vi "Storage Factory.vi"(10 "Format":T1, 11 "Config Path":path) -> (2 "Storage":refnum<class "Config Storage.lvclass">)   [LabVIEW 2020, in "VolatusConfig.lvlib"]
uses:
  VolatusConfig.lvlib
  Config Format.ctl
  lv-cdm/CDM-Config/Config Storage/Config Storage.lvclass
  lv-cdm/CDM-Config/Config-JSON/Config-JSON.lvclass
  C:/dev/lv20CE/relink/lv-cdm/CDM-Config/Config Storage/Config Storage.lvclass
  lv-cdm/CDM-Config/Config-INI/Config-INI.lvclass
  lv-cdm/CDM-Config/Config-Sqlite/Config-Sqlite.lvclass
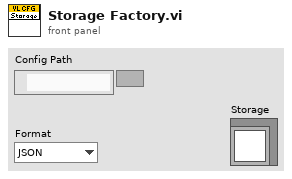
[diagram p1: front panel]
types:
  T1 = typedef "VolatusConfig.lvlib/Config Format.ctl" = enum16{"JSON", "INI", "SQLite"}
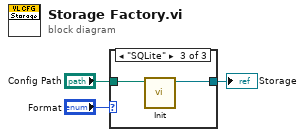
[diagram p0: block diagram]
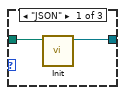
[diagram p2: hidden frame]
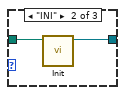
[diagram p3: hidden frame]
diagram:
  n1 = case shown="\"SQLite\"" "Format" {
    tunnel: "Config Path" -> [w5 w7 w9]
    tunnel: [w4 w6 w8] -> w1
    frame "JSON" {
      n2 = call "Init.vi"("Path"=w5) -> ("Config-JSON out"=w4:refnum<class "Config-JSON.lvclass">)  [unwired: 9 in, 1 out]
    }
    frame "INI" {
      n3 = call "Init.vi"("INI Path"=w7) -> ("Config-INI out"=w6:refnum<class "Config-INI.lvclass">)  [unwired: 9 in, 1 out]
    }
    frame "SQLite" {
      n4 = call "Init.vi"("DB Path"=w9) -> ("Config-Sqlite out"=w8:refnum<class "Config-Sqlite.lvclass">)  [unwired: 9 in, 1 out]
    }
  }
  "Storage" <- w1
